vi "VI_Generator_Generator.vi"() -> ()   [LabVIEW 2025]
uses:
  <vilib>/Utility/miscctls.llb/LVPointTypeDef.ctl
panel:
  out "Array 2":string[](array[string])
  out "unsigned byte array":u8[][](array[numeric])
  out "Loop":i32
  out "Array":string[](array[string])
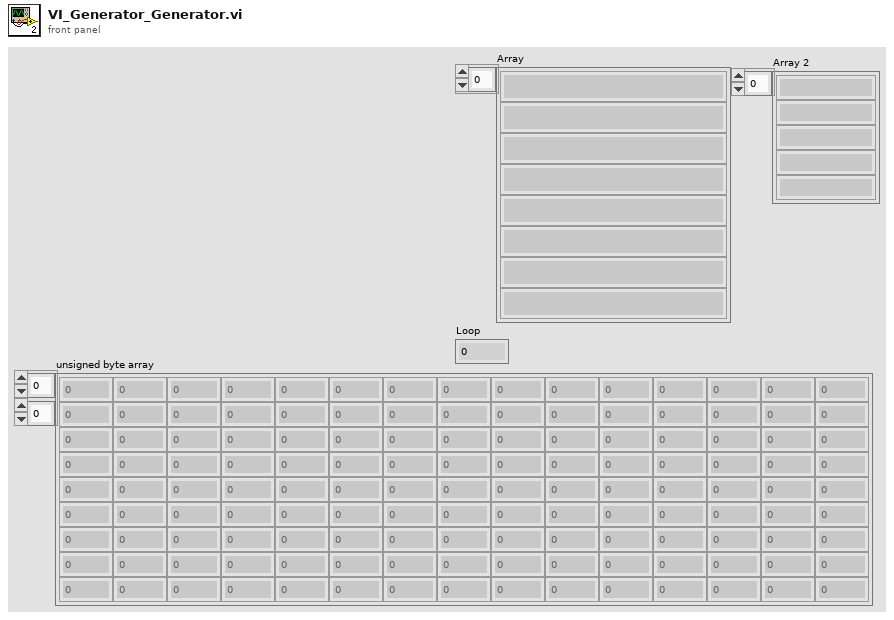
[diagram p1: front panel]
types:
  T1 = typedef "LVPointTypeDef.ctl" = cluster{"Horizontal":i16, "Vertical":i16}
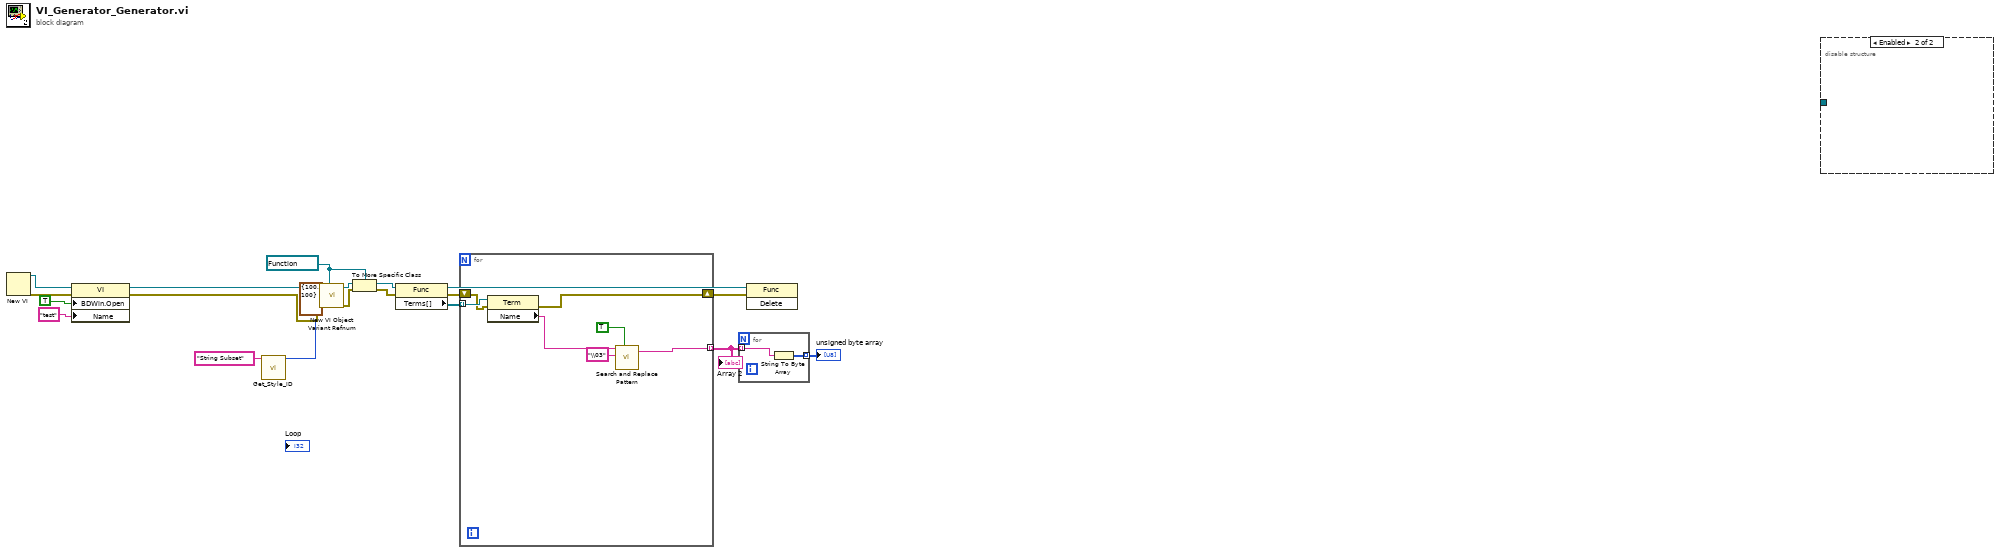
[diagram p0: block diagram]
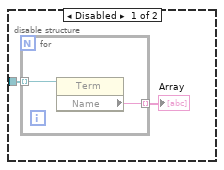
[diagram p2: hidden frame]
diagram:
  w11 = refnum<vi> refnum ("vi object class")
  n1 = New VI() -> (0:w18:errorcluster, 3:w19:refnum<vi>)  [unwired: 7 in]
  n2 = property class="VI"(reference=w19, error in=w18, "BDWin.Open"=TRUE ("Block Diagram Window:Open"), "Name"="test" ("VI Name")) -> (reference out=w16:refnum<vi>, error out=w15:errorcluster)
  n3 = call "Get_Style_ID.vi"("Style"="String Subset") -> ("style"=w4:i32)  [unwired: 8 in, 2 out]
  n4 = call "New VI Object Variant Refnum.vi"("vi object class"=w11, "error in (no error)"=w15, "location"=T1 {"Horizontal"=100, "Vertical"=100}, "style"=w4, "owner refnum"=w16) -> ("error out"=w12:errorcluster, "object refnum"=w13:refnum<vi>)  [unwired: 5 in]
  n5 = To More Specific Class(target class=w11, reference=w13, error in=w12) -> (specific class reference=w10:refnum<vi>, error out=w8:errorcluster)
  n6 = property class="Func"(reference=w10, error in=w8) -> (reference out=w6:refnum<vi>, error out=w7:errorcluster, "Terms[]"=w9:refnum<vi>[])
  n7 = for {
    tunnel: w9 -> [w27] mode=indexing
    shift-right: [w25] -> w5
    shift-left: w7 -> [w26]
    tunnel: [w23] -> w2 mode=indexing
    n8 = property class="Term"(reference=w27, error in=w26) -> (error out=w25:errorcluster, "Name"=w24:string)  [unwired: 1 out]
    n9 = call <vilib>:"Search and Replace Pattern.vi"("string"=w24, "regular expression (\"\")"="\\03" ("regular expression (\"\")"), "replace all? (F)"=TRUE) -> ("result string"=w23:string)  [unwired: 2 in, 1 out]
  }
  "Array 2" <- w2
  n10 = for {
    tunnel: w2 -> [w29] mode=indexing
    tunnel: [w28] -> w1 mode=indexing
    n11 = String To Byte Array(string=w29) -> (unsigned byte array=w28:u8[])
  }
  "unsigned byte array" <- w1
  n12 = invoke class="Func" method="Delete"(reference=w6, error in=w5) -> ()  [unwired: 1 in, 3 out]
  n13 = disable-structure shown="Enabled" {
    disable-tunnel: _ -> [w31 _]
    frame Disabled {
      n14 = for {
        tunnel: w31 -> [w33] mode=indexing
        tunnel: [w32] -> w30 mode=indexing
        n15 = property class="Term"(reference=w33) -> ("Name"=w32:string)  [unwired: 1 in, 2 out]
      }
      "Array" <- w30
    }
    frame Enabled {
    }
  }
